vi "String - Select Channel Data.vi"(10 "All Channels In":dbl[](array[numeric]), 11 "cRIO Channel List":i32[](array[numeric])) -> (2 "Selected Channel Out":dbl[](array[numeric]))   [LabVIEW 2013]
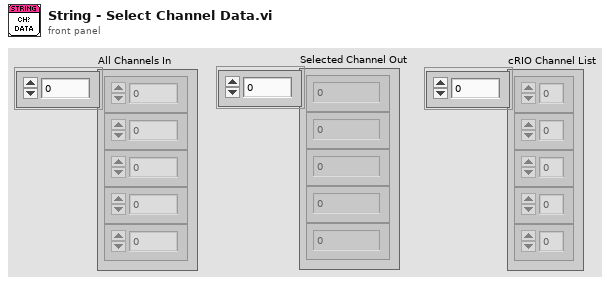
[diagram p1: front panel]
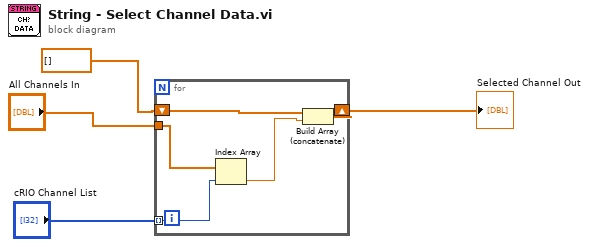
[diagram p0: block diagram]
diagram:
  n1 = for {
    shift-right: [w8] -> w4
    shift-left: dbl[] [] -> [w9]
    tunnel: "All Channels In" -> [w7]
    tunnel: "cRIO Channel List" -> [w6] mode=indexing
    n2 = Index Array(array=w7, index=w6) -> (element=w5:dbl)
    n3 = Build Array (concatenate)(w9, w5) -> (w8:dbl[])
  }
  "Selected Channel Out" <- w4
